vi "RPC Open Test App Reference.vi"(7 "port number (3363)":u16=3363, 8 "error in (no error)":errorcluster, 10 "Test ID (\"\")":string, 11 "Client (\"\": open server reference)":string) -> (0 "error out":errorcluster, 1 "Component Base Path":path, 2 "Test Component Path":path, 3 "app reference":refnum<vi>)   [LabVIEW 2011]
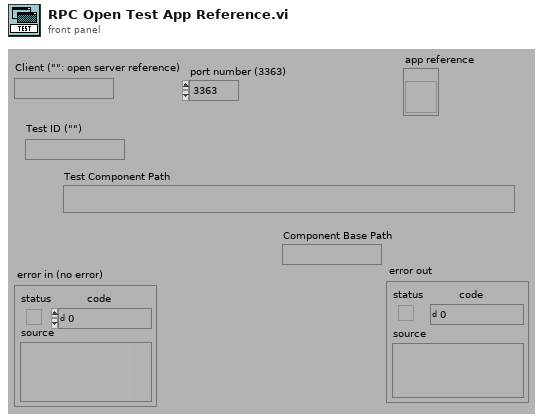
[diagram p1: front panel]
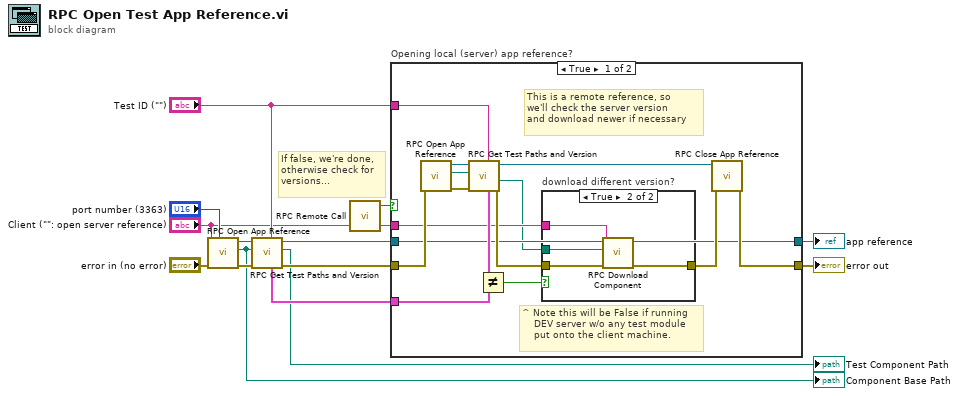
[diagram p0: block diagram]
diagram:
  # "If false, we're done,\notherwise check for\nversions..."
  n1 = call "RPC Open App Reference.vi"("Port Number (3363)"="port number (3363)", "error in (no error)"="error in (no error)", "Client (\"\": open server reference)"="Client (\"\": open server reference)") -> ("error out"=w8:errorcluster, "Component Base Path"=w5:path, "App Reference"=w10:refnum<vi>)  [unwired: 2 in, 4 out]
  "Component Base Path" <- w5
  n2 = call "RPC Get Test Paths and Version.vi"("Test ID (\"\")"="Test ID (\"\")", "error in (no error)"=w8, "Base Path (empty)"=w5, "app reference (empty)"=w10) -> ("error out"=w7:errorcluster, "Test Component Path"=→"Test Component Path":path, "app reference"=w9:refnum<vi>, "Version"=w6:cluster{"Version":string, "Build Number":u32})  [unwired: 4 out]
  n3 = call "RPC Remote Call.vi"("IP (\"\")"="Client (\"\": open server reference)") -> ("Remote Call?"=w1:bool)  [unwired: 4 out]
  n4 = case "Opening local (server) app reference?" shown="True" w1 {
    tunnel: w7 -> [w29 w35]
    tunnel: w9 -> [w17 w36]
    tunnel: [w17 w36] -> w13
    tunnel: [w26 w35] -> w12
    tunnel: "Test ID (\"\")" -> [w21 _]
    tunnel: w6 -> [w25 _]
    tunnel: "Client (\"\": open server reference)" -> [w16 _]
    frame True {
      # "^ Note this will be False if running\n    DEV server w/o any test module\n    put onto the client machine."
      # "This is a remote reference, so\nwe'll check the server version\nand download newer if necessary"
      n5 = call "RPC Open App Reference.vi"("error in (no error)"=w29) -> ("error out"=w19:errorcluster, "Component Base Path"=w22:path, "App Reference"=w24:refnum<vi>)  [unwired: 4 in, 4 out]
      n6 = call "RPC Get Test Paths and Version.vi"("Test ID (\"\")"=w21, "error in (no error)"=w19, "Base Path (empty)"=w22, "app reference (empty)"=w24) -> ("error out"=w18:errorcluster, "Test Download component"=w15:path, "app reference"=w23:refnum<vi>, "Version"=w20:cluster{"Version":string, "Build Number":u32})  [unwired: 4 out]
      n7 = Not Equal?(x=w20, y=w25) -> (x != y?=w28:bool)
      n8 = case "download different version?" shown="True" w28 {
        tunnel: w18 -> [w30 w34]
        tunnel: [w30 w33] -> w27
        tunnel: w15 -> [_ w32]
        tunnel: w16 -> [_ w31]
        frame False {
        }
        frame True {
          n9 = call "RPC Download Component.vi"("error in (no error)"=w34, "Component Path (empty)"=w32, "Client (\"\")"=w31) -> ("error out"=w33:errorcluster)  [unwired: 8 out]
        }
      }
      n10 = call "RPC Close App Reference.vi"("error in (no error)"=w27, "app reference"=w23) -> ("error out"=w26:errorcluster)  [unwired: 9 out]
    }
    frame False {
    }
  }
  "error out" <- w12
  "app reference" <- w13
